vi "LOOP_Read.vi"(4 "error in (no error)":errorcluster, 7 "connection ID":refnum<k5>) -> (0 "error out":errorcluster, 2 "LOOP response":string, 3 "connection ID out":refnum<k5>)   [LabVIEW 2025, in "CAENels FAST-PS.lvlib"]
doc: "This block performs a LOOP:? command to check the current setting of control loop mode. \nThe response is I for constant current mode and V for constant voltage mode."
uses:
  CAENels FAST-PS.lvlib
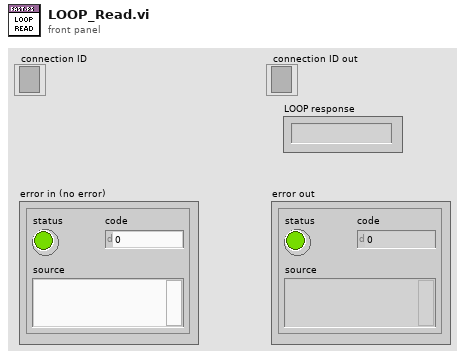
[diagram p1: front panel]
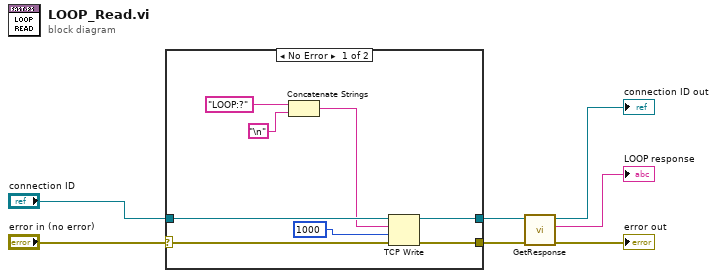
[diagram p0: block diagram]
diagram:
  n1 = case shown="No Error" "error in (no error)" {
    selector: "error in (no error)" -> [w15 w17]
    tunnel: [w14 w17] -> w3
    tunnel: [w13 w16] -> w4
    tunnel: "connection ID" -> [w12 w16]
    frame No Error {
      n2 = Concatenate Strings("LOOP:?" ("string (\"\")"), "\n") -> (w10:string)
      n3 = TCP Write(connection ID=w12, data in=w10, error in (no error)=w15, 9:1000 ("timeout ms (25000)")) -> (connection ID out=w13:refnum<k5>, error out=w14:errorcluster)  [unwired: 1 out]
    }
    frame Error {
    }
  }
  n4 = call "GetResponse.vi"("error in (no error)"=w3, "connection ID"=w4) -> ("error out"=→"error out":errorcluster, "response"=→"LOOP response":string, "connection ID out"=→"connection ID out":refnum<k5>)  [unwired: 3 in]
